vi "song+analysis.vi"() -> ()   [LabVIEW 2020]
panel:
  out "Numeric":i32
  out "Rate":dbl
  out "size(s)":i32
  out "element":waveform(dbl)
  out "Waveform Graph":waveform(dbl)[](graph)
  in  "path":path
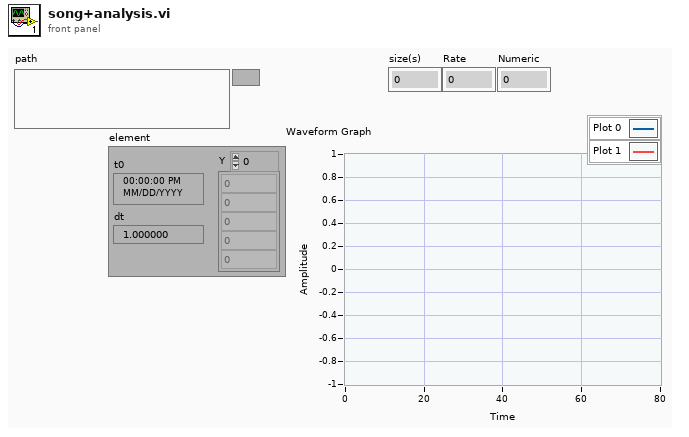
[diagram p1: front panel]
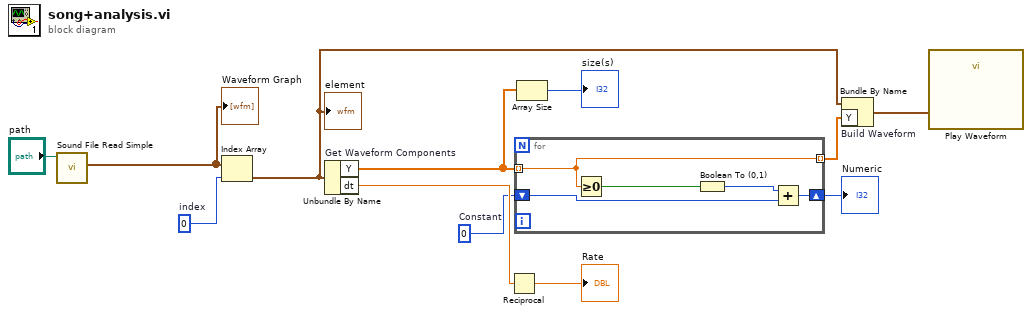
[diagram p0: block diagram]
diagram:
  w3 = 0  # Constant
  w11 = 0  # index
  n1 = call <vilib>:"Sound File Read Simple.vi"("path"="path") -> ("data"=w10:waveform(dbl)[])  [unwired: 7 in, 3 out]
  "Waveform Graph" <- w10
  n2 = Index Array "Index Array"(array=w10, index=w11) -> (element=w5:waveform(dbl))
  "element" <- w5
  n3 = Unbundle By Name "Get Waveform Components"(w5) -> ("Y"=w4:dbl[], "dt"=w8:dbl)
  n4 = Reciprocal(x=w8) -> (1/x=→"Rate":dbl)
  n5 = for {
    tunnel: w4 -> [w13] mode=indexing
    shift-right: [w15] -> w2
    shift-left: w3 -> [w16]
    tunnel: [w13] -> w1 mode=indexing
    n6 = Greater Or Equal To 0?(x=w13) -> (x >= 0?=w14:bool)
    n7 = Boolean To (0,1)(Boolean=w14) -> (0, 1=w17:i16)
    n8 = Add(x=w17, y=w16) -> (x+y=w15:i32)
  }
  "Numeric" <- w2
  n9 = Array Size(array=w4) -> (size(s)=→"size(s)":i32)
  n10 = Bundle By Name "Build Waveform"(cluster=w5, "Y"=w1) -> (w6:waveform(dbl))
  n11 = call "Play Waveform"("Data"=w6) -> ()  [unwired: 18 in, 1 out]
